vi "UpdateDisplay.vi"(7 "CmbBox Refnum":refnum<vi>, 8 "Display State In":T1 caption="State") -> ()   [LabVIEW 2009, in "HistoryPath.xctl"]
uses:
  HistoryPath.xctl
  State.ctl
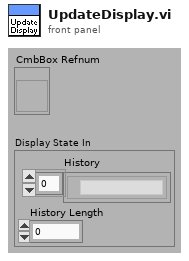
[diagram p1: front panel]
types:
  T1 = typedef "HistoryPath.xctl/State.ctl" = cluster{"History":path[], "History Length":i32}
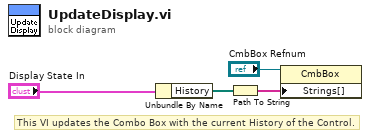
[diagram p0: block diagram]
diagram:
  # "This VI updates the Combo Box with the current History of the Control."
  n1 = Unbundle By Name("Display State In") -> ("History"=w3:path[])
  n2 = Path To String(path=w3) -> (string=w4:string[])
  n3 = property on="Property Node" class="CmbBox"(reference="CmbBox Refnum", "Strings[]"=w4) -> ()  [unwired: 1 in, 2 out]
